vi "Inject Attribute List.vi"(6 "Attributes Ref":refnum<data-value>, 8 "error in (no error)":errorcluster, 11 "Start Under Body Wash in":refnum<class "Start Under Body Wash.lvclass">) -> (0 "error out":errorcluster, 3 "Start Under Body Wash out":refnum<class "Start Under Body Wash.lvclass">)   [LabVIEW 2019, in "Start Under Body Wash.lvclass"]
uses:
  <vilib>/gpm_packages/@cs/Car-wash/Source/Process Steps/Start Under Body Wash/Start Under Body Wash.lvclass
  <vilib>/gpm_packages/@cs/lookup-table/Source/LookupTable/LookupTable.lvclass
  <vilib>/gpm_packages/@cs/lookup-table/Source/LookupTable/LookupTable.lvclass/LookupTable.ctl
  <vilib>/gpm_packages/@cs/Car-wash/Source/Process Steps/Start Under Body Wash/Start Under Body Wash.lvclass/Start Under Body Wash.ctl
  92ce1293-9ad7-4306-b513-d3b3db97d47a.vi
  <vilib>/gpm_packages/@cs/lookup-table/Source/LookupTable/Read Table Reference.vi
  92ce1293-9ad7-4306-b513-d3b3db97d47a.vi/de21dc5f-d01f-4793-99f2-b447a7373fb0.vi
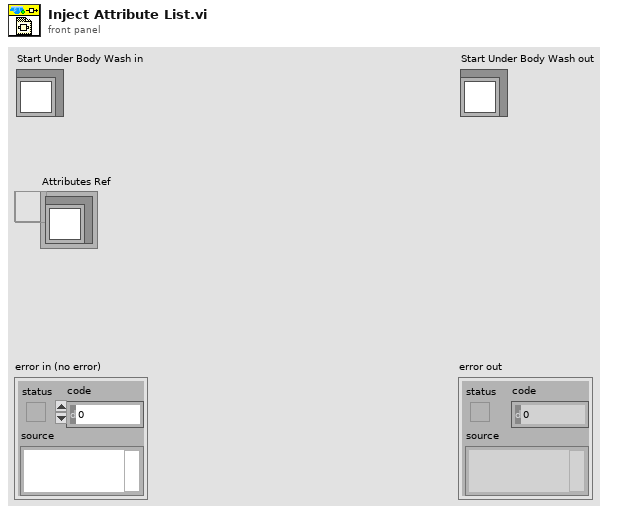
[diagram p1: front panel]
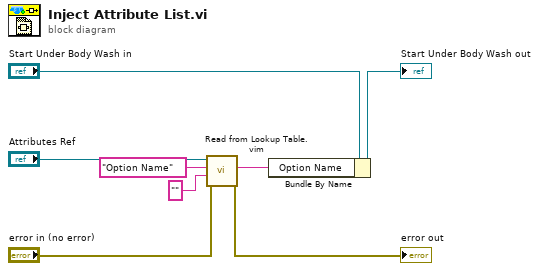
[diagram p0: block diagram]
diagram:
  n1 = call "Read from Lookup Table.vim"("error in (no error)"="error in (no error)", "Type"="", "Item Name"="Option Name", "LookupTable Reference"="Attributes Ref") -> ("error out"=→"error out":errorcluster, "Value"=w1:string)  [unwired: 4 in, 2 out]
  n2 = Bundle By Name(cluster="Start Under Body Wash in", "Option Name"=w1) -> (→"Start Under Body Wash out":refnum<class "Start Under Body Wash.lvclass">)
